vi "TemperatureDataCollection.vi"() -> ()   [LabVIEW 2022 SP3]
uses:
  <vilib>/Analysis/baseanly.llb/Mean (DBL).vi
  STOP_GLOBAL.vi
  <vilib>/Analysis/NI_AALBase.lvlib
panel:
  in  "?":enum32{"Test Firing", "Non_Important"}(tab)
  out "Temperature Data 2":dbl[](graph)
  out "Temperature Data":dynamicdata(graph)
  out "Waveform Chart":dynamicdata(graph)
  out "Temperature Data 3":dbl[](graph)
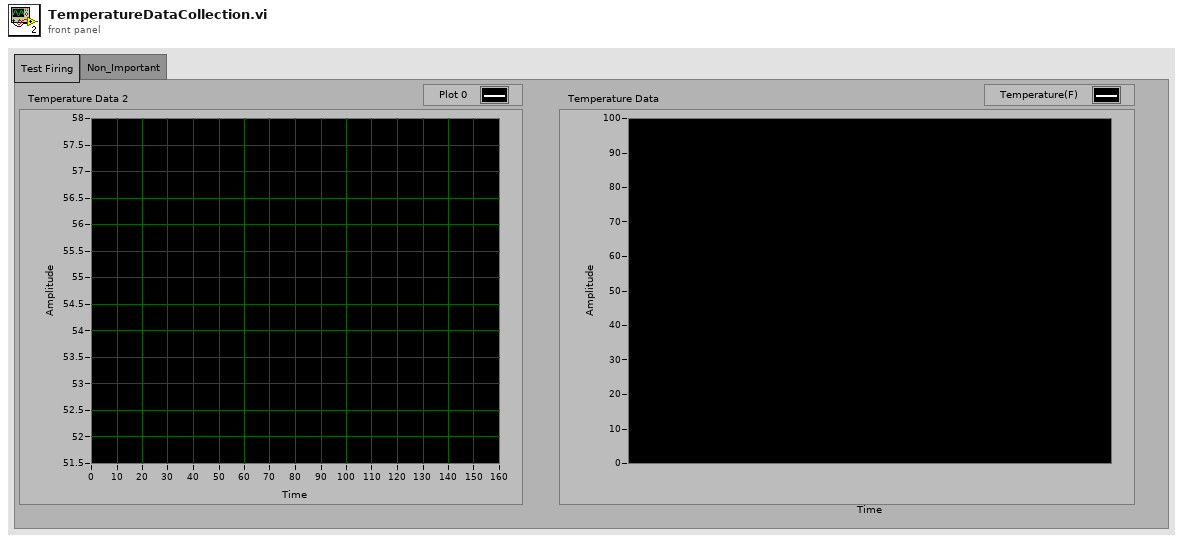
[diagram p1: front panel]
types:
  T1 = enum16{"Left Button", "Center Button", "Right Button", "Window Close"}
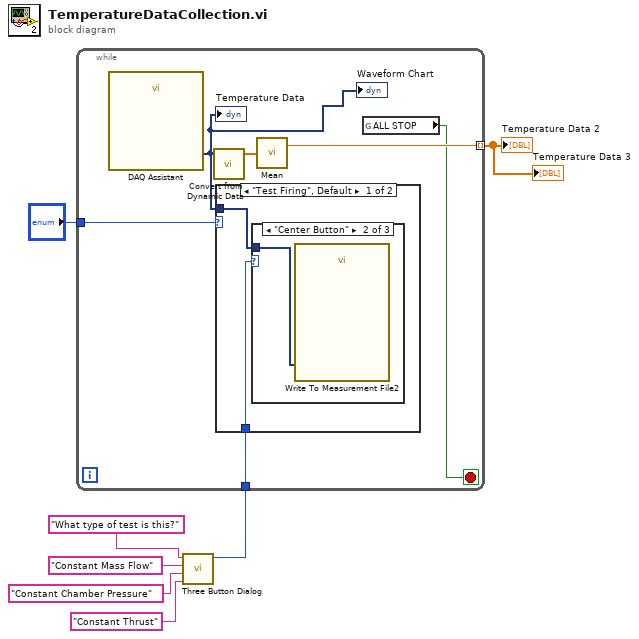
[diagram p0: block diagram]
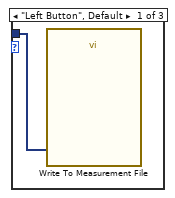
[diagram p2: hidden frame]
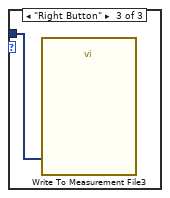
[diagram p3: hidden frame]
diagram:
  n1 = call <vilib>:"Three Button Dialog.vi"("Right Button Text (\"Cancel\")"="Constant Thrust" ("Right Button Text (\"Cancel\")"), "Center Button Text (\"No\")"="Constant Chamber Pressure" ("Center Button Text (\"No\")"), "Left Button Text (\"Yes\")"="Constant Mass Flow" ("Left Button Text (\"Yes\")"), "message"="What type of test is this?") -> ("Which Button?"=w2:T1)  [unwired: 7 in]
  n2 = while {
    tunnel: [w12] -> w1 mode=indexing
    tunnel: "?" -> [w11]
    tunnel: w2 -> [w10]
    stop <- w9 stop-if-true
    n3 = call "DAQ Assistant"() -> ("data"=w8:dynamicdata)  [unwired: 16 in, 3 out]
    "Temperature Data" <- w8
    "Waveform Chart" <- w8
    n4 = call "Convert from Dynamic Data"("Dynamic Data Type"=w8) -> ("Array"=w13:dbl[])  [unwired: 3 in]
    n5 = case shown="\"Test Firing\", Default" w11 {
      tunnel: w8 -> [w15 _]
      tunnel: w10 -> [w14 _]
      frame "Test Firing", Default {
        n6 = case shown="\"Center Button\"" w14 {
          tunnel: w15 -> [w16 w17 w18]
          frame "Left Button", Default {
            n7 = call "Write To Measurement File"("Signals"=w16) -> ()  [unwired: 16 in, 3 out]
          }
          frame "Center Button" {
            n8 = call "Write To Measurement File2"("Signals"=w17) -> ()  [unwired: 16 in, 3 out]
          }
          frame "Right Button" {
            n9 = call "Write To Measurement File3"("Signals"=w18) -> ()  [unwired: 16 in, 3 out]
          }
        }
      }
      frame "Non_Important" {
      }
    }
    n10 = call-poly <vilib>:"Mean.vi"("X"=w13) -> ("mean"=w12:dbl)  [unwired: 1 out]
    n11 = global read "STOP_GLOBAL.vi" "ALL STOP"() -> (w9:bool)
  }
  "Temperature Data 2" <- w1
  "Temperature Data 3" <- w1
